vi "超标留样启动留样.vi"(8 "error in (no error)":errorcluster) -> (0 "error out":errorcluster)   [LabVIEW 2016, in "超标留样集成.lvlib" / "德润DR803F超标留样.lvlib"]
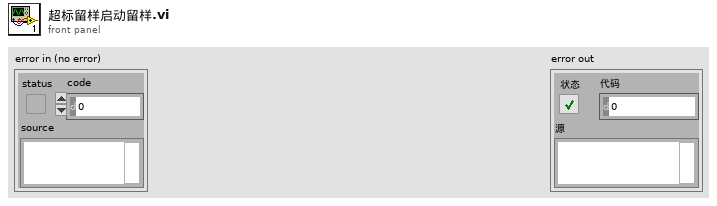
[diagram p1: front panel]
types:
  T1 = cluster{"STEP":enum16{"open", "read", "write", "close"}, "写入缓冲区":string}
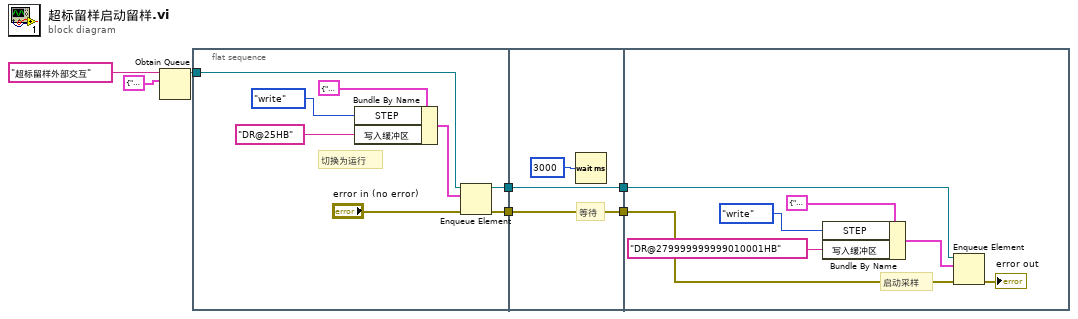
[diagram p0: block diagram]
diagram:
  n1 = Obtain Queue(name (unnamed)="超标留样外部交互" ("名称（未命名）"), element data type=T1 {"STEP"=enum."write", "写入缓冲区"="ª\u0006\u0000\u0000P`\u00000»"}) -> (queue out=w3:refnum<queue>)  [unwired: 3 in, 2 out]
  n2 = flat-sequence {
    tunnel: [w9] -> w6
    tunnel: w3 -> [w15]
    tunnel: [w8] -> w1
    tunnel: [w17] -> w7
    tunnel: w6 -> [w17]
    tunnel: [w16] -> w2
    tunnel: w1 -> [w16]
    tunnel: w7 -> [w21]
    tunnel: w2 -> [w22]
    frame #0 {
      # "切换为运行"
      n3 = Bundle By Name(cluster=T1 {"STEP"=enum."write", "写入缓冲区"="ª\u0006\u0000\u0000P`\u00000»"}, "STEP"=enum16{"open", "read", "write", "close"}."write", "写入缓冲区"="DR@25HB") -> (w10:T1)
      n4 = Enqueue Element(queue=w15, element=w10, error in (no error)="error in (no error)") -> (queue out=w8:refnum<queue>, error out=w9:errorcluster)  [unwired: 1 in, 1 out]
    }
    frame #1 {
      # "等待"
      n5 = Wait (ms)(milliseconds to wait=u32 3000 ("等待时间（毫秒）")) -> ()  [unwired: 1 out]
    }
    frame #2 {
      # "启动采样"
      n6 = Bundle By Name(cluster=T1 {"STEP"=enum."write", "写入缓冲区"="ª\u0006\u0000\u0000P`\u00000»"}, "STEP"=enum16{"open", "read", "write", "close"}."write", "写入缓冲区"="DR@279999999999010001HB") -> (w25:T1)
      n7 = Enqueue Element(queue=w22, element=w25, error in (no error)=w21) -> (error out=→"error out":errorcluster)  [unwired: 1 in, 2 out]
    }
  }
